vi "CurrentValue.vi"(11 "CurrentIn":i32) -> (3 "CurrentOut":i32)   [LabVIEW 2018]
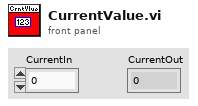
[diagram p1: front panel]
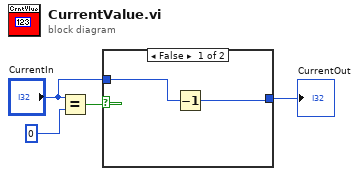
[diagram p0: block diagram]
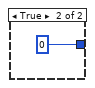
[diagram p2: hidden frame]
diagram:
  n1 = Equal?(x="CurrentIn", y=0) -> (x = y?=w3:bool)
  n2 = case shown="False" w3 {
    tunnel: [w5 0] -> w2
    tunnel: "CurrentIn" -> [w6 _]
    frame False {
      n3 = Decrement(x=w6) -> (x-1=w5:i32)
    }
    frame True {
    }
  }
  "CurrentOut" <- w2
